vi "HFRR ADV v020 new software.vi"() -> ()   [LabVIEW 2025] (continued)
    n1953 = case shown="False" w2045 {
      frame False {
      }
      frame True {
      }
    }
    n1954 = case shown="True" w2035 {
      frame False {
        n1955 = property on="Password 2" class="Str"("Visible"=FALSE) -> ()  [unwired: 2 in, 2 out]
        n1956 = local write "Password 2"("" ("Password")) -> ()
      }
      frame True {
        n1957 = property on="Password 2" class="Str"("Visible"=TRUE) -> ()  [unwired: 2 in, 2 out]
        n1958 = Equal?(x="Password 2", y="HFRR1234") -> (x = y?=w2167:bool)
        n1959 = case shown="True" w2167 {
          tunnel: "Password 2" -> [w2170 _]
          frame False {
            n1960 = String Length(string=w2170) -> (length=w2171:i32)
            n1961 = Greater Than 0?(x=w2171) -> (x > 0?=w2169:bool)
            n1962 = case shown="False" w2169 {
              frame False {
                n1963 = property on="Password 2" class="Str"("Caption.Text"="Password (Advance Setting)") -> ()  [unwired: 2 in, 2 out]
              }
              frame True {
                n1964 = property on="Password 2" class="Str"("Caption.Text"="Incorrect Password!") -> ()  [unwired: 2 in, 2 out]
              }
            }
          }
          frame True {
            n1965 = local write "EDIT 2"(FALSE ("EDIT 2")) -> ()
            n1966 = local write "Password 2"("" ("Password")) -> ()
            n1967 = local write "Main Tab"(T2."Advance" ("Main Tab")) -> ()
            n1968 = local write "Main Dashboard Buttons"(T1."Advance" ("Main Dashboard Buttons")) -> ()
          }
        }
      }
    }
    n1969 = case shown="True" "Prog Uno" {
      frame False {
      }
      frame True {
        n1970 = stacked-sequence {
          frame #0 {
            n1971 = Delete(path (use dialog)=path "C:/LAB-IQ-NXT/UNOCOMPILE.bat" ("working directory")) -> ()  [unwired: 4 in, 3 out]
          }
          frame #1 {
            n1972 = local read "Com Port 1"() -> (w2632:refnum<visa-resource-name>)
            n1973 = Concatenate Strings("cmd.exe /c \"mode " ("command line"), w2632, ":1200,n,8,1\"\n" ("command line")) -> (w2637:string)
            n1974 = Concatenate Strings(w2637, "CD\\\nCD WinDucom\navrdude -C avrdude.conf -v -patmega328p -carduino -P" ("command line"), w2632, " -b115200 -D -Uflash:w:UNO_V20.hex:i\n" ("command line"), "\r") -> (w2639:string)
            "STR" <- w2639
            n1975 = call <vilib>:"Write Characters To File.vi"("append to file? (new file:F)"=FALSE, "character string"=w2639, "file path (dialog if empty)"=path "C:/LAB-IQ/UNOCOMPILE.bat" ("working directory")) -> ()  [unwired: 2 in, 1 out]
          }
          frame #2 {
            n1976 = disable-structure shown="Disabled" {
              frame Disabled {
                w2643 = "cmd.exe  /c \"C:\\LAB-IQ-NXT\\UNOCOMPILE.bat\"" ("string")
                n1977 = local write "Prog Uno"(FALSE ("run minimized? (F)")) -> ()
                n1978 = call <vilib>:"System Exec.vi"("expected output size  (4096)"=u32 65535, "run minimized? (F)"=FALSE, "wait until completion? (T)"=TRUE ("run minimized? (F)"), "working directory"=path "C:/LAB-IQ-NXT", "standard input"=w2643, "command line"=w2643) -> ("error out"=w2642:errorcluster, "standard output"=→"String 42":string)  [unwired: 2 in, 2 out]
                "error out 3" <- w2642
                n1979 = flat-sequence {
                  tunnel: w2642 -> [_]
                  frame #0 {
                  }
                }
              }
              frame Enabled {
              }
            }
          }
        }
      }
    }
    n1980 = case shown="\"ISO 12156\"" "TEST STANDARD" {
      tunnel: [2.0 ("Set Temp") 0.0 ("Set Temp") 2.0 ("Set Temp") 0.0 ("Set Temp")] -> w2036
      frame "ASTM D6079", Default {
        w2589 = 50.0 ("Hz")
        w2590 = 53.0 ("Set Rh")
        w2592 = 1.0 ("Set Strk")
        w2591 = 60.0 ("Set Temp")
        # "astm hide"
        n1981 = local write "NORMAL LOAD"(200.0 ("NORMAL LOAD")) -> ()
        n1982 = local write "Set Strk"(w2592) -> ()
        n1983 = local write "Set Hz"(w2589) -> ()
        n1984 = local write "Set Temp"(w2591) -> ()
        n1985 = local write "Set Rh"(w2590) -> ()
        n1986 = local write "test time"(75.0 ("test time")) -> ()
        n1987 = local write "Set Stroke:"(w2592) -> ()
        n1988 = local write "Set Humidity:"(w2590) -> ()
        n1989 = local write "Set Frequency:"(w2589) -> ()
        n1990 = local write "Set Temperature:"(w2591) -> ()
        "Test Standard" <- "ASTM D6079" ("Test Standard 2")
      }
      frame "ISO 12156" {
        n1991 = local write "Set Strk"(1.0 ("Set Strk")) -> ()
        n1992 = local write "NORMAL LOAD"(200.0 ("NORMAL LOAD")) -> ()
        n1993 = local write "Set Temp"(60.0 ("Set Temp")) -> ()
        n1994 = local write "test time"(75.0 ("test time")) -> ()
        n1995 = local write "Set Hz"(50.0 ("Hz")) -> ()
        n1996 = local write "Set Rh"(53.0 ("Set Rh")) -> ()
      }
      frame "CEC F-096-A-06" {
        n1997 = local write "Set Strk"(1.0 ("Set Strk")) -> ()
        n1998 = local write "NORMAL LOAD"(200.0 ("NORMAL LOAD")) -> ()
        n1999 = local write "Set Temp"(60.0 ("Set Temp")) -> ()
        n2000 = local write "test time"(75.0 ("test time")) -> ()
        n2001 = local write "Set Hz"(50.0 ("Hz")) -> ()
        n2002 = local write "Set Rh"(53.0 ("Set Rh")) -> ()
      }
      frame "Custom" {
      }
    }
    n2003 = case shown="True" "Prog Due" {
      frame False {
      }
      frame True {
        n2004 = stacked-sequence {
          frame #0 {
            n2005 = Delete(path (use dialog)=path "C:/LAB-IQ/DUECOMPILE.bat" ("working directory")) -> ()  [unwired: 4 in, 3 out]
          }
          frame #1 {
            n2006 = disable-structure shown="Disabled" {
              frame Disabled {
                n2007 = local read "visa due"() -> (w2614:string)
                n2008 = Concatenate Strings("cmd.exe /c \"mode " ("command line"), w2614, ":1200,n,8,1\"\n" ("command line")) -> (w2619:string)
                n2009 = Concatenate Strings(w2619, "CD\\\nCD WinDucom\nTIMEOUT 1\n bossac.exe -i -d --port=" ("command line"), w2614, " -U false -e -w -v -b DUE.bin -R\n" ("command line"), "\r") -> (w2621:string)
                "concatenated string 2" <- w2621
                n2010 = call <vilib>:"Write Characters To File.vi"("append to file? (new file:F)"=FALSE, "character string"=w2621, "file path (dialog if empty)"=path "C:/LAB-IQ-NXT/DUECOMPILE.bat" ("working directory")) -> ()  [unwired: 2 in, 1 out]
              }
              frame Enabled {
              }
            }
          }
          frame #2 {
            # "C:\\LAB-IQ-NXT\\DUECOMPILE.bat"
            n2011 = disable-structure shown="Disabled" {
              frame Disabled {
                w2626 = "cmd.exe  /c \"C:\\LAB-IQ-NXT\\DUECOMPILE.bat\"" ("string")
                n2012 = call <vilib>:"System Exec.vi"("expected output size  (4096)"=u32 65535, "run minimized? (F)"=FALSE, "wait until completion? (T)"=TRUE ("run minimized? (F)"), "working directory"=path "C:/LAB-IQ-NXT", "standard input"=w2626, "command line"=w2626) -> ("error out"=w2625:errorcluster, "standard output"=→"String 44":string)  [unwired: 2 in, 2 out]
                "error out 4" <- w2625
                n2013 = flat-sequence {
                  tunnel: w2625 -> [_]
                  frame #0 {
                  }
                }
              }
              frame Enabled {
              }
            }
            n2014 = local write "Prog Due"(FALSE ("Prog Due")) -> ()
          }
        }
      }
    }
    n2015 = Or(x=w2033, y=w2031) -> (x .or. y?=w2032:bool)
    n2016 = case shown="\"About\"" w2030 {
      tunnel: [T27."Acquire" ("Main Tab") T27."Compare Files" ("Main Tab") T27."About" ("Main Tab")] -> w2043
      frame "Acquire", Default {
      }
      frame "Compare Files" {
      }
      frame "About" {
      }
    }
    n2017 = Or(x=w2037, y="OPEN") -> (x .or. y?=w2038:bool)
    n2018 = case shown="True" w2038 {
      tunnel: w2037 -> [_ w2178]
      frame False {
      }
      frame True {
        n2019 = stacked-sequence {
          tunnel: w2178 -> [_ w2245 _ _]
          frame #0 {
            w2194 = "  " ("String 6")
            n2020 = local write "OPEN"(FALSE ("open")) -> ()
            n2021 = local read "string1 2"() -> (w2182:string)
            n2022 = local read "string1 3"() -> (w2181:string)
            n2023 = local read "string1 4"() -> (w2180:string)
            n2024 = property on="OPEN" class="Bool (strict)"("Visible"=FALSE) -> ()  [unwired: 2 in, 2 out]
            n2025 = local write "String 6"(w2194) -> ()
            n2026 = local write "String 7"(w2194) -> ()
            n2027 = local write "String 8"(w2194) -> ()
            n2028 = local write "String 12"(w2194) -> ()
            n2029 = local read "OK Button 16"() -> (w2179:bool)
            n2030 = String To Path(string=w2182) -> (path=w2190:path)
            n2031 = String To Path(string=w2181) -> (path=w2189:path)
            n2032 = String To Path(string=w2180) -> (path=w2188:path)
            n2033 = case shown="True" w2179 {
              tunnel: [w2195 w2196] -> w2183
              frame False {
                n2034 = local read "string1"() -> (w2195:string)
              }
              frame True {
                n2035 = local read "String Indicator 4"() -> (w2196:string)
              }
            }
            n2036 = Open/Create/Replace File "Open File"(file path (use dialog)=w2190) -> (refnum out=w2186:refnum<file>)  [unwired: 5 in, 2 out]
            n2037 = Open/Create/Replace File "Open File"(file path (use dialog)=w2189) -> (refnum out=w2185:refnum<file>)  [unwired: 5 in, 2 out]
            n2038 = Open/Create/Replace File "Open File"(file path (use dialog)=w2188) -> (refnum out=w2184:refnum<file>)  [unwired: 5 in, 2 out]
            n2039 = while {
              tunnel: w2186 -> [w2208]
              i -> [w2204]
              stop <- w2203 continue-if-true
              (unwired) TRUE ("line mode (F)")
              n2040 = Read from Text File "Read File"(file (use dialog)=w2208) -> (text=w2205:string)  [unwired: 3 in, 3 out]
              n2041 = local write "Numeric 11"(w2204) -> ()
              n2042 = String Length(string=w2205) -> (length=w2207:i32)
              n2043 = Greater?(x=w2207, y=1) -> (0:w2203:bool)
            }
            n2044 = while {
              tunnel: w2185 -> [w2214]
              i -> [w2210]
              stop <- w2209 continue-if-true
              (unwired) TRUE ("line mode (F)")
              n2045 = Read from Text File "Read File"(file (use dialog)=w2214) -> (text=w2211:string)  [unwired: 3 in, 3 out]
              n2046 = local write "Numeric 12"(w2210) -> ()
              n2047 = String Length(string=w2211) -> (length=w2213:i32)
              n2048 = Greater?(x=w2213, y=1) -> (0:w2209:bool)
            }
            n2049 = while {
              tunnel: w2184 -> [w2220]
              i -> [w2216]
              stop <- w2215 continue-if-true
              (unwired) TRUE ("line mode (F)")
              n2050 = Read from Text File "Read File"(file (use dialog)=w2220) -> (text=w2217:string)  [unwired: 3 in, 3 out]
              n2051 = local write "Numeric 13"(w2216) -> ()
              n2052 = String Length(string=w2217) -> (length=w2219:i32)
              n2053 = Greater?(x=w2219, y=1) -> (0:w2215:bool)
            }
            n2054 = String To Path(string=w2183) -> (path=w2191:path)
            n2055 = Open/Create/Replace File "Open File"(file path (use dialog)=w2191) -> (refnum out=w2187:refnum<file>)  [unwired: 5 in, 2 out]
            n2056 = while {
              tunnel: w2187 -> [w2202]
              i -> [w2198]
              stop <- w2197 continue-if-true
              (unwired) TRUE ("line mode (F)")
              n2057 = Read from Text File "Read File"(file (use dialog)=w2202) -> (text=w2199:string)  [unwired: 3 in, 3 out]
              n2058 = local write "Numeric 8"(w2198) -> ()
              n2059 = String Length(string=w2199) -> (length=w2201:i32)
              n2060 = Greater?(x=w2201, y=1) -> (0:w2197:bool)
            }
          }
          frame #1 {
            w2372 = FALSE ("ACTUAL   MERGE")
            # "Sample Temp"
            # "ECR"
            # "COF"
            # "Time\nCOF\nFF\nTemp"
            n2061 = case shown="True" w2245 {
              tunnel: [w2392 w2393] -> w2246
              frame False {
                n2062 = local read "string1"() -> (w2392:string)
              }
              frame True {
                n2063 = local read "String Indicator 4"() -> (w2393:string)
              }
            }
            n2064 = local read "string1 3"() -> (w2290:string)
            n2065 = String To Path(string=w2246) -> (path=w2377:path)
            n2066 = String To Path(string=w2290) -> (path=w2388:path)
            n2067 = local read "Numeric 12"() -> (w2374:i32)
            n2068 = local read "Numeric 8"() -> (w2376:i32)
            n2069 = local read "string1 2"() -> (w2291:string)
            n2070 = local read "string1 4"() -> (w2289:string)
            n2071 = Open/Create/Replace File "Open File"(file path (use dialog)=w2377) -> (refnum out=w2391:refnum<file>, error out=w2390:errorcluster)  [unwired: 5 in, 1 out]
            n2072 = Open/Create/Replace File "Open File"(file path (use dialog)=w2388) -> (refnum out=w2384:refnum<file>, error out=w2385:errorcluster)  [unwired: 5 in, 1 out]
            n2073 = for {
              N: w2376 -> [_]
              tunnel: w2391 -> [w2539]
              tunnel: w2390 -> [w2538]
              tunnel: [w2528] -> w2303 mode=indexing
              tunnel: [w2526] -> w2360 mode=indexing
              tunnel: [w2527] -> w2355 mode=indexing
              tunnel: w2372 -> [_]
              tunnel: [w2520] -> w2357 mode=indexing
              tunnel: [w2516] -> w2326 mode=indexing
              tunnel: [w2512] -> w2301 mode=indexing
              tunnel: [w2508] -> w2282 mode=indexing
              tunnel: [w2503] -> w2242 mode=indexing
              (unwired) TRUE ("line mode (F)")
              # "freq"
              # "Stroke"
              # "Time"
              # "CoF"
              # "Humidity"
              # "Temp"
              # "Air Temp"
              # "ECR"
              n2074 = Read from Text File "Read File"(file (use dialog)=w2539, error in=w2538) -> (text=w2504:string)  [unwired: 2 in, 3 out]
              n2075 = local write "String 6"(w2504) -> ()
              n2076 = String Subset(string=w2504, offset (0)=0, length (rest)=14 ("length (rest)")) -> (substring=w2532:string)
              n2077 = String Subset(string=w2504, offset (0)=35, length (rest)=9 ("length (rest)")) -> (substring=w2529:string)
              n2078 = String Subset(string=w2504, offset (0)=15, length (rest)=9 ("length (rest)")) -> (substring=w2535:string)
              n2079 = Fract/Exp String To Number(string=w2532) -> (number=w2528:dbl)  [unwired: 3 in, 1 out]
              n2080 = Fract/Exp String To Number(string=w2529) -> (number=w2527:dbl)  [unwired: 3 in, 1 out]
              n2081 = Fract/Exp String To Number(string=w2535) -> (number=w2526:dbl)  [unwired: 3 in, 1 out]
              n2082 = String Subset(string=w2504, offset (0)=85, length (rest)=9 ("length (rest)")) -> (substring=w2505:string)
              n2083 = String Subset(string=w2504, offset (0)=25, length (rest)=9 ("length (rest)")) -> (substring=w2511:string)
              n2084 = String Subset(string=w2504, offset (0)=55, length (rest)=9 ("length (rest)")) -> (substring=w2513:string)
              n2085 = String Subset(string=w2504, offset (0)=45, length (rest)=9 ("length (rest)")) -> (substring=w2519:string)
              n2086 = String Subset(string=w2504, offset (0)=65, length (rest)=9 ("length (rest)")) -> (substring=w2525:string)
              n2087 = Fract/Exp String To Number(string=w2511) -> (number=w2508:dbl)  [unwired: 3 in, 1 out]
              n2088 = Fract/Exp String To Number(string=w2505) -> (number=w2503:dbl)  [unwired: 3 in, 1 out]
              n2089 = Fract/Exp String To Number(string=w2513) -> (number=w2512:dbl)  [unwired: 3 in, 1 out]
              n2090 = Fract/Exp String To Number(string=w2519) -> (number=w2516:dbl)  [unwired: 3 in, 1 out]
              n2091 = Fract/Exp String To Number(string=w2525) -> (number=w2522:dbl)  [unwired: 3 in, 1 out]
              n2092 = Add(x=w2522, y=0.0) -> (x+y=w2520:dbl)
            }
            n2093 = for {
              N: w2374 -> [_]
              tunnel: w2385 -> [w2465]
              tunnel: w2384 -> [w2464]
              tunnel: [w2454] -> w2343 mode=indexing
              tunnel: [w2452] -> w2341 mode=indexing
              tunnel: [w2453] -> w2337 mode=indexing
              tunnel: w2372 -> [_]
              tunnel: [w2446] -> w2339 mode=indexing
              tunnel: [w2442] -> w2321 mode=indexing
              tunnel: [w2438] -> w2297 mode=indexing
              tunnel: [w2435] -> w2278 mode=indexing
              tunnel: [w2431] -> w2237 mode=indexing
              (unwired) 9 ("length (rest)")
              (unwired) 9 ("length (rest)")
              (unwired) TRUE ("line mode (F)")
              n2094 = Read from Text File "Read File"(file (use dialog)=w2464, error in=w2465) -> (text=w2432:string)  [unwired: 2 in, 3 out]
              n2095 = local write "String 8"(w2432) -> ()
              n2096 = String Subset(string=w2432, offset (0)=85) -> (substring=w2434:string)  [unwired: 1 in]
              n2097 = String Subset(string=w2432, offset (0)=35, length (rest)=9 ("length (rest)")) -> (substring=w2455:string)
              n2098 = String Subset(string=w2432, offset (0)=55, length (rest)=9 ("length (rest)")) -> (substring=w2440:string)
              n2099 = String Subset(string=w2432, offset (0)=25) -> (substring=w2436:string)  [unwired: 1 in]
              n2100 = String Subset(string=w2432, offset (0)=15, length (rest)=9 ("length (rest)")) -> (substring=w2461:string)
              n2101 = String Subset(string=w2432, offset (0)=0, length (rest)=14 ("length (rest)")) -> (substring=w2458:string)
              n2102 = String Subset(string=w2432, offset (0)=45, length (rest)=9 ("length (rest)")) -> (substring=w2445:string)
              n2103 = String Subset(string=w2432, offset (0)=65, length (rest)=9 ("length (rest)")) -> (substring=w2451:string)
              n2104 = Fract/Exp String To Number(string=w2434) -> (number=w2431:dbl)  [unwired: 3 in, 1 out]
              n2105 = Fract/Exp String To Number(string=w2455) -> (number=w2453:dbl)  [unwired: 3 in, 1 out]
              n2106 = Fract/Exp String To Number(string=w2440) -> (number=w2438:dbl)  [unwired: 3 in, 1 out]
              n2107 = Fract/Exp String To Number(string=w2436) -> (number=w2435:dbl)  [unwired: 3 in, 1 out]
              n2108 = Fract/Exp String To Number(string=w2461) -> (number=w2452:dbl)  [unwired: 3 in, 1 out]
              n2109 = Fract/Exp String To Number(string=w2458) -> (number=w2454:dbl)  [unwired: 3 in, 1 out]
              n2110 = Fract/Exp String To Number(string=w2445) -> (number=w2442:dbl)  [unwired: 3 in, 1 out]
              n2111 = Fract/Exp String To Number(string=w2451) -> (number=w2448:dbl)  [unwired: 3 in, 1 out]
              n2112 = Add(x=w2448, y=0.0) -> (x+y=w2446:dbl)
            }
            n2113 = String To Path(string=w2291) -> (path=w2389:path)
            n2114 = String To Path(string=w2289) -> (path=w2383:path)
            n2115 = local read "Numeric 11"() -> (w2373:i32)
            n2116 = local read "Numeric 13"() -> (w2375:i32)
            n2117 = Open/Create/Replace File "Open File"(file path (use dialog)=w2389) -> (refnum out=w2387:refnum<file>, error out=w2386:errorcluster)  [unwired: 5 in, 1 out]
            n2118 = Open/Create/Replace File "Open File"(file path (use dialog)=w2383) -> (refnum out=w2382:refnum<file>, error out=w2381:errorcluster)  [unwired: 5 in, 1 out]
            n2119 = for {
              N: w2373 -> [_]
              tunnel: w2387 -> [w2502]
              tunnel: w2386 -> [w2501]
              tunnel: [w2491] -> w2353 mode=indexing
              tunnel: [w2489] -> w2351 mode=indexing
              tunnel: [w2490] -> w2346 mode=indexing
              tunnel: w2372 -> [_]
              tunnel: [w2483] -> w2348 mode=indexing
              tunnel: [w2479] -> w2324 mode=indexing
              tunnel: [w2475] -> w2299 mode=indexing
              tunnel: [w2471] -> w2280 mode=indexing
              tunnel: [w2466] -> w2238 mode=indexing
              (unwired) TRUE ("line mode (F)")
              n2120 = Read from Text File "Read File"(file (use dialog)=w2502, error in=w2501) -> (text=w2467:string)  [unwired: 2 in, 3 out]
              n2121 = local write "String 7"(w2467) -> ()
              n2122 = String Subset(string=w2467, offset (0)=85, length (rest)=9 ("length (rest)")) -> (substring=w2470:string)
              n2123 = String Subset(string=w2467, offset (0)=35, length (rest)=9 ("length (rest)")) -> (substring=w2492:string)
              n2124 = String Subset(string=w2467, offset (0)=55, length (rest)=9 ("length (rest)")) -> (substring=w2478:string)
              n2125 = String Subset(string=w2467, offset (0)=25, length (rest)=9 ("length (rest)")) -> (substring=w2472:string)
              n2126 = String Subset(string=w2467, offset (0)=45, length (rest)=9 ("length (rest)")) -> (substring=w2480:string)
              n2127 = String Subset(string=w2467, offset (0)=0, length (rest)=14 ("length (rest)")) -> (substring=w2495:string)
              n2128 = String Subset(string=w2467, offset (0)=15, length (rest)=9 ("length (rest)")) -> (substring=w2498:string)
              n2129 = String Subset(string=w2467, offset (0)=65, length (rest)=9 ("length (rest)")) -> (substring=w2484:string)
              n2130 = Fract/Exp String To Number(string=w2470) -> (number=w2466:dbl)  [unwired: 3 in, 1 out]
              n2131 = Fract/Exp String To Number(string=w2492) -> (number=w2490:dbl)  [unwired: 3 in, 1 out]
              n2132 = Fract/Exp String To Number(string=w2478) -> (number=w2475:dbl)  [unwired: 3 in, 1 out]
              n2133 = Fract/Exp String To Number(string=w2472) -> (number=w2471:dbl)  [unwired: 3 in, 1 out]
              n2134 = Fract/Exp String To Number(string=w2480) -> (number=w2479:dbl)  [unwired: 3 in, 1 out]
              n2135 = Fract/Exp String To Number(string=w2495) -> (number=w2491:dbl)  [unwired: 3 in, 1 out]
              n2136 = Fract/Exp String To Number(string=w2498) -> (number=w2489:dbl)  [unwired: 3 in, 1 out]
              n2137 = Fract/Exp String To Number(string=w2484) -> (number=w2487:dbl)  [unwired: 3 in, 1 out]
              n2138 = Add(x=w2487, y=0.0) -> (x+y=w2483:dbl)
            }
            n2139 = for {
              N: w2375 -> [_]
              tunnel: w2382 -> [w2430]
              tunnel: w2381 -> [w2429]
              tunnel: [w2419] -> w2335 mode=indexing
              tunnel: [w2418] -> w2328 mode=indexing
              tunnel: w2372 -> [_]
              tunnel: [w2407] -> w2333 mode=indexing
              tunnel: [w2412] -> w2330 mode=indexing
              tunnel: [w2408] -> w2320 mode=indexing
              tunnel: [w2403] -> w2295 mode=indexing
              tunnel: [w2399] -> w2276 mode=indexing
              tunnel: [w2394] -> w2236 mode=indexing
              (unwired) 1.0 ("x")
              (unwired) TRUE ("line mode (F)")
              n2140 = Read from Text File "Read File"(file (use dialog)=w2430, error in=w2429) -> (text=w2395:string)  [unwired: 2 in, 3 out]
              n2141 = local write "String 12"(w2395) -> ()
              n2142 = String Subset(string=w2395, offset (0)=85, length (rest)=9 ("length (rest)")) -> (substring=w2397:string)
              n2143 = String Subset(string=w2395, offset (0)=35, length (rest)=9 ("length (rest)")) -> (substring=w2420:string)
              n2144 = String Subset(string=w2395, offset (0)=55, length (rest)=9 ("length (rest)")) -> (substring=w2405:string)
              n2145 = String Subset(string=w2395, offset (0)=25, length (rest)=9 ("length (rest)")) -> (substring=w2401:string)
              n2146 = String Subset(string=w2395, offset (0)=45, length (rest)=9 ("length (rest)")) -> (substring=w2410:string)
              n2147 = String Subset(string=w2395, offset (0)=15, length (rest)=9 ("length (rest)")) -> (substring=w2426:string)
              n2148 = String Subset(string=w2395, offset (0)=0, length (rest)=14 ("length (rest)")) -> (substring=w2423:string)
              n2149 = String Subset(string=w2395, offset (0)=65, length (rest)=9 ("length (rest)")) -> (substring=w2413:string)
              n2150 = Fract/Exp String To Number(string=w2397) -> (number=w2394:dbl)  [unwired: 3 in, 1 out]
              n2151 = Fract/Exp String To Number(string=w2420) -> (number=w2418:dbl)  [unwired: 3 in, 1 out]
              n2152 = Fract/Exp String To Number(string=w2405) -> (number=w2403:dbl)  [unwired: 3 in, 1 out]
              n2153 = Fract/Exp String To Number(string=w2401) -> (number=w2399:dbl)  [unwired: 3 in, 1 out]
              n2154 = Fract/Exp String To Number(string=w2410) -> (number=w2408:dbl)  [unwired: 3 in, 1 out]
              n2155 = Fract/Exp String To Number(string=w2426) -> (number=w2407:dbl)  [unwired: 3 in, 1 out]
              n2156 = Fract/Exp String To Number(string=w2423) -> (number=w2419:dbl)  [unwired: 3 in, 1 out]
              n2157 = Fract/Exp String To Number(string=w2413) -> (number=w2416:dbl)  [unwired: 3 in, 1 out]
              n2158 = Add(x=w2416, y=0.0) -> (x+y=w2412:dbl)
            }
            n2159 = Delete From Array(array=w2278, index=0) -> (array with subset deleted=w2251:dbl[])  [unwired: 1 in, 1 out]
            n2160 = Delete From Array(array=w2341, index=0) -> (array with subset deleted=w2314:dbl[])  [unwired: 1 in, 1 out]
            n2161 = Delete From Array(array=w2321, index=0) -> (array with subset deleted=w2309:dbl[])  [unwired: 1 in, 1 out]
            n2162 = Delete From Array(array=w2339, index=0) -> (array with subset deleted=w2340:dbl[])  [unwired: 1 in, 1 out]
            n2163 = call-poly <vilib>:"Mean.vi"("X"=w2251) -> ("mean"=→"КОФ2 4":dbl)  [unwired: 1 out]
            n2164 = call-poly <vilib>:"Mean.vi"("X"=w2314) -> ("mean"=→"КОФ3":dbl)  [unwired: 1 out]
            n2165 = call-poly <vilib>:"Mean.vi"("X"=w2309) -> ("mean"=→"CP3":dbl)  [unwired: 1 out]
            n2166 = Delete From Array(array=w2303, index=0) -> (array with subset deleted=w2230:dbl[])  [unwired: 1 in, 1 out]
            n2167 = Delete From Array(array=w2242, index=0) -> (array with subset deleted=w2229:dbl[])  [unwired: 1 in, 1 out]
            n2168 = Delete From Array(array=w2282, index=0) -> (array with subset deleted=w2253:dbl[])  [unwired: 1 in, 1 out]
            n2169 = Delete From Array(array=w2360, index=0) -> (array with subset deleted=w2315:dbl[])  [unwired: 1 in, 1 out]
            n2170 = Delete From Array(array=w2326, index=0) -> (array with subset deleted=w2311:dbl[])  [unwired: 1 in, 1 out]
            "array w/ subset deleted" <- w2311
            n2171 = Delete From Array(array=w2357, index=0) -> (array with subset deleted=w2358:dbl[])  [unwired: 1 in, 1 out]
            n2172 = call-poly <vilib>:"Mean.vi"("X"=w2253) -> ("mean"=→"КОФ2 2":dbl)  [unwired: 1 out]
            n2173 = call-poly <vilib>:"Mean.vi"("X"=w2315) -> ("mean"=→"КОФ1":dbl)  [unwired: 1 out]
            n2174 = Bundle "Bundle"(w2230, w2229) -> (w2235:cluster{dbl[], dbl[]})  [unwired: 1 in]
            n2175 = Bundle "Bundle"(w2230, w2358) -> (w2222:cluster{dbl[], dbl[]})  [unwired: 1 in]
            n2176 = Delete From Array(array=w2237, index=0) -> (array with subset deleted=w2225:dbl[])  [unwired: 1 in, 1 out]
            n2177 = Delete From Array(array=w2238, index=0) -> (array with subset deleted=w2227:dbl[])  [unwired: 1 in, 1 out]
            n2178 = Delete From Array(array=w2348, index=0) -> (array with subset deleted=w2349:dbl[])  [unwired: 1 in, 1 out]
            n2179 = Delete From Array(array=w2236, index=0) -> (array with subset deleted=w2223:dbl[])  [unwired: 1 in, 1 out]
            n2180 = Delete From Array(array=w2330, index=0) -> (array with subset deleted=w2331:dbl[])  [unwired: 1 in, 1 out]
            n2181 = Delete From Array(array=w2355, index=0) -> (array with subset deleted=w2261:dbl[])  [unwired: 1 in, 1 out]
            n2182 = Delete From Array(array=w2301, index=0) -> (array with subset deleted=w2257:dbl[])  [unwired: 1 in, 1 out]
            n2183 = Delete From Array(array=w2337, index=0) -> (array with subset deleted=w2259:dbl[])  [unwired: 1 in, 1 out]
            n2184 = Delete From Array(array=w2297, index=0) -> (array with subset deleted=w2255:dbl[])  [unwired: 1 in, 1 out]
            n2185 = Delete From Array(array=w2346, index=0) -> (array with subset deleted=w2260:dbl[])  [unwired: 1 in, 1 out]
            n2186 = Delete From Array(array=w2299, index=0) -> (array with subset deleted=w2256:dbl[])  [unwired: 1 in, 1 out]
            n2187 = Delete From Array(array=w2280, index=0) -> (array with subset deleted=w2252:dbl[])  [unwired: 1 in, 1 out]
            n2188 = Delete From Array(array=w2324, index=0) -> (array with subset deleted=w2310:dbl[])  [unwired: 1 in, 1 out]
            n2189 = Delete From Array(array=w2351, index=0) -> (array with subset deleted=w2312:dbl[])  [unwired: 1 in, 1 out]
            n2190 = Delete From Array(array=w2328, index=0) -> (array with subset deleted=w2258:dbl[])  [unwired: 1 in, 1 out]
            n2191 = Delete From Array(array=w2295, index=0) -> (array with subset deleted=w2254:dbl[])  [unwired: 1 in, 1 out]
            n2192 = Delete From Array(array=w2276, index=0) -> (array with subset deleted=w2250:dbl[])  [unwired: 1 in, 1 out]
            n2193 = Delete From Array(array=w2320, index=0) -> (array with subset deleted=w2308:dbl[])  [unwired: 1 in, 1 out]
            n2194 = Delete From Array(array=w2333, index=0) -> (array with subset deleted=w2313:dbl[])  [unwired: 1 in, 1 out]
            n2195 = Delete From Array(array=w2343, index=0) -> (array with subset deleted=w2226:dbl[])  [unwired: 1 in, 1 out]
            n2196 = Delete From Array(array=w2353, index=0) -> (array with subset deleted=w2228:dbl[])  [unwired: 1 in, 1 out]
            n2197 = Delete From Array(array=w2335, index=0) -> (array with subset deleted=w2224:dbl[])  [unwired: 1 in, 1 out]
            n2198 = Bundle "Bundle"(w2230, w2261) -> (w2248:cluster{dbl[], dbl[]})  [unwired: 1 in]
            n2199 = Bundle "Bundle"(w2230, w2315) -> (w2249:cluster{dbl[], dbl[]})  [unwired: 1 in]
            n2200 = Bundle "Bundle"(w2261, w2257) -> (w2263:cluster{dbl[], dbl[]})  [unwired: 1 in]
            n2201 = Bundle "Bundle"(w2226, w2225) -> (w2233:cluster{dbl[], dbl[]})  [unwired: 1 in]
            n2202 = Bundle "Bundle"(w2259, w2255) -> (w2265:cluster{dbl[], dbl[]})  [unwired: 1 in]
            n2203 = Bundle "Bundle"(w2226, w2259) -> (w2369:cluster{dbl[], dbl[]})  [unwired: 1 in]
            n2204 = Bundle "Bundle"(w2226, w2255) -> (w2293:cluster{dbl[], dbl[]})  [unwired: 1 in]
            n2205 = Bundle "Bundle"(w2226, w2314) -> (w2379:cluster{dbl[], dbl[]})  [unwired: 1 in]
            n2206 = Bundle "Bundle"(w2226, w2309) -> (w2317:cluster{dbl[], dbl[]})  [unwired: 1 in]
            n2207 = Bundle "Bundle"(w2226, w2340) -> (w2364:cluster{dbl[], dbl[]})  [unwired: 1 in]
            n2208 = Bundle "Bundle"(w2260, w2256) -> (w2264:cluster{dbl[], dbl[]})  [unwired: 1 in]
            n2209 = Bundle "Bundle"(w2228, w2227) -> (w2234:cluster{dbl[], dbl[]})  [unwired: 1 in]
            n2210 = Bundle "Bundle"(w2228, w2260) -> (w2371:cluster{dbl[], dbl[]})  [unwired: 1 in]
            n2211 = Bundle "Bundle"(w2228, w2256) -> (w2294:cluster{dbl[], dbl[]})  [unwired: 1 in]
            n2212 = Bundle "Bundle"(w2228, w2310) -> (w2318:cluster{dbl[], dbl[]})  [unwired: 1 in]
            n2213 = Bundle "Bundle"(w2228, w2312) -> (w2380:cluster{dbl[], dbl[]})  [unwired: 1 in]
            n2214 = Bundle "Bundle"(w2228, w2349) -> (w2362:cluster{dbl[], dbl[]})  [unwired: 1 in]
            n2215 = Bundle "Bundle"(w2258, w2254) -> (w2266:cluster{dbl[], dbl[]})  [unwired: 1 in]
            n2216 = Bundle "Bundle"(w2224, w2223) -> (w2232:cluster{dbl[], dbl[]})  [unwired: 1 in]
            n2217 = Bundle "Bundle"(w2224, w2258) -> (w2370:cluster{dbl[], dbl[]})  [unwired: 1 in]
            n2218 = Bundle "Bundle"(w2224, w2254) -> (w2292:cluster{dbl[], dbl[]})  [unwired: 1 in]
            n2219 = Bundle "Bundle"(w2224, w2308) -> (w2316:cluster{dbl[], dbl[]})  [unwired: 1 in]
            n2220 = Bundle "Bundle"(w2224, w2313) -> (w2378:cluster{dbl[], dbl[]})  [unwired: 1 in]
            n2221 = Bundle "Bundle"(w2224, w2331) -> (w2363:cluster{dbl[], dbl[]})  [unwired: 1 in]
            n2222 = call-poly <vilib>:"Mean.vi"("X"=w2311) -> ("mean"=→"CP1":dbl)  [unwired: 1 out]
            n2223 = call-poly <vilib>:"Mean.vi"("X"=w2252) -> ("mean"=→"КОФ2 3":dbl)  [unwired: 1 out]
            n2224 = call-poly <vilib>:"Mean.vi"("X"=w2310) -> ("mean"=→"CP2":dbl)  [unwired: 1 out]
            n2225 = call-poly <vilib>:"Mean.vi"("X"=w2312) -> ("mean"=→"КОФ2":dbl)  [unwired: 1 out]
            n2226 = call-poly <vilib>:"Mean.vi"("X"=w2250) -> ("mean"=→"КОФ2 5":dbl)  [unwired: 1 out]
            n2227 = call-poly <vilib>:"Mean.vi"("X"=w2308) -> ("mean"=→"CP4":dbl)  [unwired: 1 out]
            n2228 = call-poly <vilib>:"Mean.vi"("X"=w2313) -> ("mean"=→"КОФ4":dbl)  [unwired: 1 out]
            n2229 = Bundle "Bundle"(w2230, w2257) -> (w2221:cluster{dbl[], dbl[]})  [unwired: 1 in]
            n2230 = Bundle "Bundle"(w2230, w2311) -> (w2244:cluster{dbl[], dbl[]})  [unwired: 1 in]
            n2231 = Build Array "Build Array"(w2221, w2244) -> (w2247:cluster{dbl[], dbl[]}[])
            "XY Graph 17" <- w2247
            n2232 = Build Array "Build Array"(w2235, w2234, w2233, w2232) -> (→"Frequency ( Hz )":cluster{dbl[], dbl[]}[])
            n2233 = Build Array "Build Array"(w2263, w2264, w2265, w2266) -> (→"Air Temp ( °C ) vs Humidity ( % RH )":cluster{dbl[], dbl[]}[])
            n2234 = Build Array "Build Array"(w2248, w2371, w2369, w2370) -> (→"Air Temperature  ( °C )":cluster{dbl[], dbl[]}[])
            n2235 = Build Array "Build Array"(w2221, w2294, w2293, w2292) -> (→"Humidity ( %RH )":cluster{dbl[], dbl[]}[])
            n2236 = Build Array "Build Array"(w2249, w2380, w2379, w2378) -> (→"Coefficient Of Friction":cluster{dbl[], dbl[]}[])
            n2237 = Build Array "Build Array"(w2244, w2318, w2317, w2316) -> (→"Sample Temperature ( °C )":cluster{dbl[], dbl[]}[])
            n2238 = Build Array "Build Array"(w2222, w2362, w2364, w2363) -> (→"XY Graph 13":cluster{dbl[], dbl[]}[])
            n2239 = Bundle "Bundle"(w2230, w2253) -> (w2275:cluster{dbl[], dbl[]})  [unwired: 1 in]
            n2240 = Bundle "Bundle"(w2226, w2251) -> (w2273:cluster{dbl[], dbl[]})  [unwired: 1 in]
            n2241 = Bundle "Bundle"(w2228, w2252) -> (w2274:cluster{dbl[], dbl[]})  [unwired: 1 in]
            n2242 = Bundle "Bundle"(w2224, w2250) -> (w2272:cluster{dbl[], dbl[]})  [unwired: 1 in]
            n2243 = Build Array "Build Array"(w2275, w2274, w2273, w2272) -> (→"Stroke ( mm )":cluster{dbl[], dbl[]}[])
            n2244 = local write "XY Graph 16"(w2247) -> ()
          }
          frame #2 {
          }
          frame #3 {
            n2245 = local write "Numeric 8"(0 ("Numeric 8")) -> ()
            n2246 = local write "Numeric 11"(0 ("Numeric 11")) -> ()
            n2247 = local write "Numeric 12"(0 ("Numeric 12")) -> ()
            n2248 = local write "Numeric 13"(0 ("Numeric 13")) -> ()
            n2249 = property on="OPEN" class="Bool (strict)"("Visible"=TRUE) -> ()  [unwired: 2 in, 2 out]
            n2250 = local read "String Control 2"() -> (w2547:string)
            n2251 = local read "String Control 4"() -> (w2546:string)
            n2252 = local read "String Control 6"() -> (w2545:string)
            n2253 = local read "String Control 8"() -> (w2544:string)
            n2254 = Match Pattern(string=w2547, regular expression="Samples / cycle :- ") -> (after substring=w2561:string)  [unwired: 1 in, 3 out]
            n2255 = Match Pattern(string=w2547, regular expression="Frequency :- ") -> (after substring=w2580:string)  [unwired: 1 in, 3 out]
            n2256 = Match Pattern(string=w2546, regular expression="Samples / cycle :- ") -> (after substring=w2557:string)  [unwired: 1 in, 3 out]
            n2257 = Match Pattern(string=w2546, regular expression="Frequency :- ") -> (after substring=w2575:string)  [unwired: 1 in, 3 out]
            n2258 = Match Pattern(string=w2545, regular expression="Samples / cycle :- ") -> (after substring=w2553:string)  [unwired: 1 in, 3 out]
            n2259 = Match Pattern(string=w2545, regular expression="Frequency :- ") -> (after substring=w2570:string)  [unwired: 1 in, 3 out]
            n2260 = Match Pattern(string=w2544, regular expression="Samples / cycle :- ") -> (after substring=w2549:string)  [unwired: 1 in, 3 out]
            n2261 = Match Pattern(string=w2544, regular expression="Frequency :- ") -> (after substring=w2565:string)  [unwired: 1 in, 3 out]
            n2262 = String Subset(string=w2561, length (rest)=6 ("length (rest)")) -> (substring=w2563:string)  [unwired: 1 in]
            n2263 = String Subset(string=w2580, length (rest)=9 ("length (rest)")) -> (substring=w2582:string)  [unwired: 1 in]
            n2264 = String Subset(string=w2557, length (rest)=6 ("length (rest)")) -> (substring=w2559:string)  [unwired: 1 in]
            n2265 = String Subset(string=w2575, length (rest)=9 ("length (rest)")) -> (substring=w2577:string)  [unwired: 1 in]
            n2266 = String Subset(string=w2553, length (rest)=6 ("length (rest)")) -> (substring=w2555:string)  [unwired: 1 in]
            n2267 = String Subset(string=w2570, length (rest)=9 ("length (rest)")) -> (substring=w2572:string)  [unwired: 1 in]
            n2268 = String Subset(string=w2549, length (rest)=6 ("length (rest)")) -> (substring=w2551:string)  [unwired: 1 in]
            n2269 = String Subset(string=w2565, length (rest)=9 ("length (rest)")) -> (substring=w2567:string)  [unwired: 1 in]
            n2270 = Fract/Exp String To Number(string=w2563) -> (number=w2543:dbl)  [unwired: 3 in, 1 out]
            n2271 = Fract/Exp String To Number(string=w2582) -> (number=w2583:dbl)  [unwired: 3 in, 1 out]
            n2272 = Fract/Exp String To Number(string=w2559) -> (number=w2542:dbl)  [unwired: 3 in, 1 out]
            n2273 = Fract/Exp String To Number(string=w2577) -> (number=w2578:dbl)  [unwired: 3 in, 1 out]
            n2274 = Fract/Exp String To Number(string=w2555) -> (number=w2541:dbl)  [unwired: 3 in, 1 out]
            n2275 = Fract/Exp String To Number(string=w2572) -> (number=w2573:dbl)  [unwired: 3 in, 1 out]
            n2276 = Fract/Exp String To Number(string=w2551) -> (number=w2540:dbl)  [unwired: 3 in, 1 out]
            n2277 = Fract/Exp String To Number(string=w2567) -> (number=w2568:dbl)  [unwired: 3 in, 1 out]
            n2278 = local write "sample1"(w2543) -> ()
            n2279 = local write "freq1"(w2583) -> ()
            n2280 = local write "sample2"(w2542) -> ()
            n2281 = local write "freq2"(w2578) -> ()
            n2282 = local write "sample3"(w2541) -> ()
            n2283 = local write "freq3"(w2573) -> ()
            n2284 = local write "sample4"(w2540) -> ()
            n2285 = local write "freq 4"(w2568) -> ()
          }
        }
      }
    }
    n2286 = case shown="True" w2032 {
      selector: w2032 -> [_ w2160]
      frame False {
      }
      frame True {
        n2287 = Not(x=w2160) -> (.not. x?=w2156:bool)
        n2288 = local write "service 3"(w2156) -> ()
        n2289 = local write "OPEN 6"(w2156) -> ()
        n2290 = call <vilib>:"System Exec.vi"("wait until completion? (T)"=TRUE, "command line"="C:\\LAB-IQ\\Scar View.exe") -> ("error out"=→"error out 5":errorcluster)  [unwired: 6 in, 3 out]
      }
    }
    n2291 = case shown="\"Acquire\", Default" w2043 {
      frame "Acquire", Default {
        w3056 = 0.2 ("y")
        w3061 = 1.0 ("y")
        w3062 = 0.8 ("y")
        # "Elapsed time\ncof\nstroke\nAir temp\nTemp\nHumidity"
        n2292 = disable-structure shown="Disabled" {
          frame Disabled {
            n2293 = local read "Flag"() -> (w3079:dbl)
            n2294 = local read "RUN"() -> (w3076:bool)
            n2295 = Not(x=w3076) -> (.not. x?=w3075:bool)
            n2296 = Equal?(x=w3079, y=10.0) -> (x = y?=w3077:bool)
            n2297 = And(x=w3077, y=w3075) -> (x .and. y?=w3074:bool)
            n2298 = case shown="True" w3074 {
              frame False {
              }
              frame True {
                w3080 = FALSE ("Heater Button")
                n2299 = local write "Humidity"(w3080) -> ()
                n2300 = local write "Heater Button"(w3080) -> ()
              }
            }
          }
          frame Enabled {
          }
        }
        n2301 = disable-structure shown="Disabled" {
          frame Disabled {
            n2302 = case shown="True" {
              selector: _ -> [_ _]
              frame False {
              }
              frame True {
                w3171 = TRUE ("Heater")
                n2303 = local write "Humidity"(w3171) -> ()
                n2304 = local write "Heater Button"(w3171) -> ()
                n2305 = local read "TEST STANDARD"() -> (w3174:T3)
                n2306 = local read "TEST STANDARD"() -> (w3169:T3)
                n2307 = Equal?(x=w3174, y=enum16{"ASTM D6079", "ISO 12156", "Custom"}."ISO 12156" ("Test Standard")) -> (x = y?=w3172:bool)
                n2308 = Equal?(x=w3169, y=enum16{"ASTM D6079", "ISO 12156", "Custom"}."ASTM D6079" ("Test Standard")) -> (x = y?=w3168:bool)
                n2309 = case shown="True" w3172 {
                  frame False {
                  }
                  frame True {
                    n2310 = local write "Heater"(TRUE ("Heater")) -> ()
                    n2311 = local write "airtempflg"(FALSE ("airtempflg")) -> ()
                  }
                }
                n2312 = case shown="True" w3168 {
                  frame False {
                  }
                  frame True {
                    n2313 = local write "Heater"(FALSE ("Heater")) -> ()
                    n2314 = local write "airtempflg"(TRUE ("airtempflg")) -> ()
                  }
                }
              }
            }
          }
          frame Enabled {
          }
        }
        n2315 = stacked-sequence {
          frame #0 {
            n2316 = case shown="True" "RST FF" {
              frame False {
              }
              frame True {
                w3237 = 0.0 ("X Scale.Range:Maximum")
                n2317 = property on="Frictional Force ( N )" class="WFChart (strict)"("XScale.Maximum"=600.0 ("X Scale.Range:Maximum"), "XScale.Minimum"=w3237, "YScale.Maximum"=10.0 ("Y Scale.Range:Maximum"), "YScale.Minimum"=w3237) -> ()  [unwired: 2 in, 2 out]
              }
            }
          }
          frame #1 {
            n2318 = case shown="True" "RST TEMP" {
              frame False {
              }
              frame True {
                n2319 = property on="Temperature ( Deg C )" class="WFChart (strict)"("XScale.Minimum"=0.0 ("X Scale.Range:Minimum"), "XScale.Maximum"=600.0 ("X Scale.Range:Maximum"), "YScale.Minimum"=0.0 ("Y Scale.Range:Minimum"), "YScale.Maximum"=100.0 ("Y Scale.Range:Maximum")) -> ()  [unwired: 2 in, 2 out]
              }
            }
          }
          frame #2 {
            n2320 = case shown="True" "RSTCOF" {
              frame False {
              }
              frame True {
                n2321 = property on="Coefficient of Friction" class="WFChart (strict)"("XScale.Minimum"=0.0 ("X Scale.Range:Minimum"), "XScale.Maximum"=600.0 ("X Scale.Range:Maximum"), "YScale.Maximum"=1.0 ("X Scale.Range:Minimum"), "YScale.Minimum"=0.0 ("X Scale.Range:Minimum")) -> ()  [unwired: 2 in, 2 out]
              }
            }
          }
          frame #3 {
            n2322 = case shown="True" "RSTCOF 2" {
              frame False {
              }
              frame True {
                (unwired) 100.0 ("Y Scale.Range:Maximum")
                (unwired) 0.0 ("Y Scale.Range:Minimum")
                (unwired) 600.0 ("X Scale.Range:Maximum")
                (unwired) 0.0 ("X Scale.Range:Minimum")
              }
            }
          }
          frame #4 {
            n2323 = case shown="True" "RSTCOF 3" {
              frame False {
              }
              frame True {
                n2324 = property on="Electrical Contact Resistance ( % )" class="WFChart (strict)"("XScale.Minimum"=0.0 ("X Scale.Range:Minimum"), "XScale.Maximum"=600.0 ("X Scale.Range:Maximum"), "YScale.Minimum"=0.0 ("Y Scale.Range:Minimum"), "YScale.Maximum"=100.0 ("Y Scale.Range:Maximum")) -> ()  [unwired: 2 in, 2 out]
              }
            }
          }
        }
        n2325 = disable-structure shown="Disabled" {
          frame Disabled {
            n2326 = case shown="True" {
              selector: _ -> [_ _]
              frame False {
              }
              frame True {
                n2327 = local read "zflag 2"() -> (w3138:dbl)
                n2328 = local read "yflag"() -> (w3140:dbl)
                n2329 = Equal?(x=w3140, y=2.0 ("tflag")) -> (x = y?=w3142:bool)
                n2330 = Equal?(x=w3138, y=3.0 ("tflag")) -> (x = y?=w3141:bool)
                n2331 = And(x=w3142, y=w3141) -> (x .and. y?=w3136:bool)
                n2332 = case shown="True" w3136 {
                  frame False {
                  }
                  frame True {
                    w3167 = 0.0 ("zflag")
                    n2333 = local write "zflag"(w3167) -> ()
                    n2334 = local write "zflag 2"(w3167) -> ()
                    n2335 = Delete(path (use dialog)=path "C:/LAB-IQ-NXT/WO 2449 TT.sig" ("file path (dialog if empty)")) -> (deleted path=w3166:path)  [unwired: 4 in, 2 out]
                    n2336 = Delete(path (use dialog)=path "C:/LAB-IQ-NXT/WO 2449 TRH.sig" ("file path (dialog if empty)")) -> (deleted path=w3161:path)  [unwired: 4 in, 2 out]
                    n2337 = local read "SEN.RUN HRS"() -> (w3153:dbl)
                    n2338 = local read "SENSOR TIME"() -> (w3151:dbl)
                    n2339 = call <vilib>:"compatOverwrite.vi"("overwrite (F)"=TRUE) -> ("overwrite?"=w3143:T30)
                    n2340 = call <vilib>:"compatOverwrite.vi"("overwrite (F)"=TRUE) -> ("overwrite?"=w3147:T30)
                    n2341 = local read "Total No. of Tests"() -> (w3154:dbl)
                    n2342 = Add(x=w3151, y=w3153) -> (x+y=w3152:dbl)
                    "SEN.RUN HRS" <- w3152
                    n2343 = Open/Create/Replace File(file path (use dialog)=w3166, operation (0:open)=w3143) -> (refnum out=w3144:refnum<file>, error out=w3145:errorcluster)  [unwired: 4 in, 1 out]
                    n2344 = Open/Create/Replace File(file path (use dialog)=w3161, operation (0:open)=w3147) -> (refnum out=w3148:refnum<file>, error out=w3149:errorcluster)  [unwired: 4 in, 1 out]
                    n2345 = Deny Access(4:w3145, 6:T28."deny none" ("deny mode (2)"), 7:w3144) -> (3:w3165:refnum<file>)  [unwired: 1 out]
                    n2346 = Deny Access(4:w3149, 6:T28."deny none" ("deny mode (2)"), 7:w3148) -> (3:w3157:refnum<file>)  [unwired: 1 out]
                    n2347 = Number To Decimal String(number=w3154) -> (decimal integer string=w3162:string)  [unwired: 1 in]
                    n2348 = Number To Decimal String(number=w3152) -> (decimal integer string=w3158:string)  [unwired: 1 in]
                    n2349 = Write to Binary File(file (use dialog)=w3165, data=w3162, 5:FALSE ("prepend array or string size? (T)")) -> ()  [unwired: 3 in, 3 out]
                    n2350 = Write to Binary File(file (use dialog)=w3157, data=w3158, 5:FALSE ("prepend array or string size? (T)")) -> ()  [unwired: 3 in, 3 out]
                  }
                }
              }
            }
          }
          frame Enabled {
          }
        }
        n2351 = local read "RUN"() -> (w3065:bool)
        n2352 = local read "run replace"() -> (w3069:bool)
        n2353 = local read "run replace"() -> (w3068:bool)
        n2354 = case shown="True" w3065 {
          frame False {
            n2355 = local write "run replace"(FALSE ("run replace")) -> ()
          }
          frame True {
            "run replace" <- TRUE ("run replace")
          }
        }
        n2356 = local read "RUN"() -> (w3073:bool)
        n2357 = local read "Set Temp"() -> (w3035:dbl)
        n2358 = local read "SetTemp"() -> (w3037:dbl)
        n2359 = case shown="False" w3073 {
          tunnel: [FALSE ("TEST RUNNING") TRUE ("TEST RUNNING")] -> w3072
          frame False {
            w3256 = 0.0 ("Flag")
            n2360 = local write "Elapsed time"(0.0 ("elapsedtime")) -> ()
            n2361 = local write "Time Remaining"(w3256) -> ()
            n2362 = local write "Flag"(w3256) -> ()
            n2363 = local write "Remaining Time"(w3256) -> ()
          }
          frame True {
            n2364 = local write "Flag"(10.0 ("Flag")) -> ()
          }
        }
        n2365 = case shown="False" w3069 {
          frame False {
            n2366 = local read "zflag"() -> (→"zflag 2":dbl)
            n2367 = local write "yflag"(2.0 ("tflag")) -> ()
            n2368 = local write "FLAG 4"(0.0 ("FLAG")) -> ()
          }
          frame True {
            n2369 = local write "yflag"(1.0 ("tflag")) -> ()
            n2370 = local write "zflag"(3.0 ("zflag")) -> ()
          }
        }
        n2371 = local read "acq 2"() -> (w3067:bool)
        n2372 = local read "AIR TEMP"() -> (w3030:dbl)
        n2373 = local read "Amb temp"() -> (w3034:dbl)
        n2374 = case shown="True" "Save & Continue" {
          frame False {
          }
          frame True {
            "acq 2" <- TRUE ("acq 2")
          }
        }
        n2375 = local read "Set Rh"() -> (w3036:dbl)
        n2376 = Add(x=w3037, y=w3062) -> (x+y=w3063:dbl)
        n2377 = Subtract(x=w3037, y=w3062) -> (x-y=w3064:dbl)
        n2378 = Add(x=w3035, y=w3056) -> (x+y=w3057:dbl)
        n2379 = Subtract(x=w3035, y=w3056) -> (x-y=w3058:dbl)
        n2380 = And(x=w3067, y=w3068) -> (x .and. y?=w3066:bool)
        n2381 = Greater Or Equal?(x=w3030, y=15.0) -> (x >= y?=w3031:bool)
        "powstat" <- w3031
        n2382 = local read "Humidity ( %RH )"() -> (w3033:dbl)
        n2383 = case shown="True" "Save & Continue" {
          frame False {
          }
          frame True {
            n2384 = while {
              tunnel: "0123456789abcdefghijklmnopqrstuvwxyzABCDEFGHIJKLMNOPQRSTUVWXYZ" ("string 2") -> [w3227]
              shift-right: [w3225] -> w3220
              shift-left: "" -> [w3224]
              i -> [w3234]
              stop <- w3233 stop-if-true
              n2385 = Random Number (0-1)() -> (number: 0 to 1=w3228:dbl)
              n2386 = Multiply(x=w3228, y=62.0) -> (x*y=w3230:dbl)
              n2387 = Decrement(x="Length") -> (x-1=w3223:i16)
              n2388 = To Word Integer(number=w3230) -> (16bit integer=w3231:i16)
              n2389 = String Subset(string=w3227, offset (0)=w3231, length (rest)=1 ("length (rest)")) -> (substring=w3226:string)
              n2390 = Greater Or Equal?(x=w3234, y=w3223) -> (x >= y?=w3233:bool)
              n2391 = Concatenate Strings(w3226, w3224) -> (w3225:string)
            }
            n2392 = local write "UUID"(w3220) -> ()
          }
        }
        n2393 = In Range and Coerce(upper limit=w3063, x=w3034, lower limit=w3064) -> (In Range?=w3053:bool)  [unwired: 1 out]
        n2394 = Add(x=w3036, y=w3061) -> (x+y=w3060:dbl)
        n2395 = Subtract(x=w3036, y=w3061) -> (x-y=w3059:dbl)
        n2396 = local read "TEMP"() -> (w3032:dbl)
        n2397 = case shown="True" "Save & Continue" {
          frame False {
          }
          frame True {
            n2398 = local read "Operator ID"() -> (w3551:string)
            n2399 = local read "FILE"() -> (w3557:string)
            n2400 = String Length(string=w3557) -> (length=w3555:i32)
            n2401 = String Length(string=w3551) -> (length=w3552:i32)
            n2402 = Greater?(x=w3555, y=0) -> (0:w3554:bool)
            n2403 = Greater?(x=w3552, y=0) -> (0:w3550:bool)
            n2404 = And(x=w3554, y=w3550) -> (x .and. y?=w3549:bool)
            n2405 = case shown="True" w3549 {
              frame False {
                n2406 = stacked-sequence {
                  frame #0 {
                    n2407 = One Button Dialog(message="Please Enter a File Name and Operator ID to save data !", button name ("OK")="Ok") -> ()  [unwired: 1 out]
                  }
                  frame #1 {
                    n2408 = local write "Save & Continue"(FALSE ("OK Button")) -> ()
                  }
                }
                n2409 = local write "Save & Continue"(FALSE ("OK Button")) -> ()
              }
              frame True {
                n2410 = stacked-sequence {
                  frame #0 {
                    n2411 = local read "FILE"() -> (w3563:string)
                    n2412 = call "file check.vi"("file name in"=w3563) -> ("file name out"=w3562:string)  [unwired: 9 in, 1 out]
                    n2413 = call <vilib>:"Application Directory.vi"() -> ("Application Directory"=w3573:path)
                    n2414 = Build Path(base path=w3573, name or relative path="data") -> (appended path=w3572:path)
                    n2415 = call <vilib>:"Trim Whitespace.vi"("string"=w3562) -> ("trimmed string"=w3570:string)  [unwired: 1 in]
                    n2416 = call <vilib>:"Trim Whitespace.vi"("string"=w3562) -> ("trimmed string"=w3571:string)  [unwired: 1 in]
                    n2417 = List Folder(path=w3572) -> (folder names=w3568:string[])  [unwired: 3 in, 3 out]
                    n2418 = Match Pattern(string=w3570, regular expression="_(") -> (before substring=w3567:string)  [unwired: 1 in, 3 out]
                    n2419 = for {
                      tunnel: w3568 -> [w3582] mode=indexing
                      tunnel: w3567 -> [w3580]
                      shift-right: [w3578] -> w3565
                      shift-left: bool[] [] -> [w3579]
                      n2420 = Match Pattern(string=w3582, regular expression="_(") -> (before substring=w3581:string)  [unwired: 1 in, 3 out]
                      n2421 = Equal?(x=w3581, y=w3580) -> (x = y?=w3577:bool)
                      n2422 = case shown="True" w3577 {
                        tunnel: w3577 -> [_ w3585]
                        tunnel: w3579 -> [w3584 w3587]
                        tunnel: [w3584 w3586] -> w3578
                        frame False {
                        }
                        frame True {
                          n2423 = Insert Into Array(array=w3587, new element=w3585) -> (w3586:bool[])  [unwired: 1 in]
                        }
                      }
                    }
                    n2424 = Equal?(x=w3568, y=w3567) -> (x = y?=w3576:bool[])
                    n2425 = Or Array Elements(Boolean array=w3576) -> (logical OR=w3575:bool)
                    n2426 = Array Size(array=w3565) -> (size(s)=w3564:i32)
                    n2427 = case shown="True" w3575 {
                      tunnel: w3571 -> [_ w3595]
                      tunnel: w3564 -> [_ w3588]
                      frame False {
                      }
                      frame True {
                        n2428 = Number To Decimal String(number=w3588) -> (decimal integer string=w3591:string)  [unwired: 1 in]
                        n2429 = Search/Split String(string=w3595, search string/char (-)="_(" ("regular expression")) -> (substring before match=w3593:string)  [unwired: 1 in, 2 out]
                        n2430 = Concatenate Strings(w3593, "_(" ("regular expression"), w3591, ")" ("regular expression")) -> (w3589:string)
                        n2431 = local write "FILE"(w3589) -> ()
                      }
                    }
                  }
                  frame #1 {
                    w3597 = 0.0
                    w3610 = cluster{"y":dbl, dbl, "y":dbl}[] [] ("History Data")
                    w3611 = FALSE ("Heater Button")
                    (unwired) ")!" ("string")
                    (unwired) ")" ("string")
                    w3609 = dbl[] [] ("History Data")
                    w3615 = "\r"
                    # "C:\\WinDucom\\Data\\"
                    # "C:\\LAB-IQ-NXT\\data"
                    n2432 = local write "Humidity ( %RH )"(w3597) -> ()
                    n2433 = local write "Frequency ( Hz )"(w3597) -> ()
                    n2434 = local write "Stroke 3"(w3597) -> ()
                    n2435 = local write "speedop"(0.0 ("PIDclk 2")) -> ()
                    n2436 = local write "Set Temp 2"(65.0 ("Set Temp 2")) -> ()
                    n2437 = local write "AIR TEMP"(w3597) -> ()
                    n2438 = local write "clk"(0.0 ("clk")) -> ()
                    n2439 = local write "Stroke 4"(w3597) -> ()
                    n2440 = local write "COF 2"(w3597) -> ()
                    n2441 = local write "TEMP"(w3597) -> ()
                    n2442 = local write "ecr 3"(w3597) -> ()
                    n2443 = local write "FF 3"(w3597) -> ()
                    n2444 = local write "FF 2"(w3597) -> ()
                    n2445 = property on="Humidity ( %RH )" class="WFChart (strict)"("History Data"=w3609) -> ()  [unwired: 2 in, 2 out]
                    n2446 = property on="Coefficient of Friction" class="WFChart (strict)"("History Data"=w3609) -> ()  [unwired: 2 in, 2 out]
                    n2447 = property on="Coefficient of Friction" class="WFChart (strict)"("History Data"=w3609) -> ()  [unwired: 2 in, 2 out]
                    n2448 = property on="Frictional Force ( N )" class="WFChart (strict)"("History Data"=w3609) -> ()  [unwired: 2 in, 2 out]
                    n2449 = property on="Electrical Contact Resistance ( % )" class="WFChart (strict)"("History Data"=w3609) -> ()  [unwired: 2 in, 2 out]
                    n2450 = property on="Electrical Contact Resistance ( % )" class="WFChart (strict)"("History Data"=w3609) -> ()  [unwired: 2 in, 2 out]
                    n2451 = property on="Temperature ( Deg C )" class="WFChart (strict)"("History Data"=w3609) -> ()  [unwired: 2 in, 2 out]
                    n2452 = property on="Frictional Force ( N )" class="WFChart (strict)"("History Data"=w3609) -> ()  [unwired: 2 in, 2 out]
                    n2453 = property on="Coefficient of Friction" class="WFChart (strict)"("History Data"=w3609) -> ()  [unwired: 2 in, 2 out]
                    n2454 = property on="Frictional Force ( N )" class="WFChart (strict)"("History Data"=w3609) -> ()  [unwired: 2 in, 2 out]
                    n2455 = property on="Electrical Contact Resistance ( % )" class="WFChart (strict)"("History Data"=w3609) -> ()  [unwired: 2 in, 2 out]
                    n2456 = property on="Temperature ( Deg C )" class="WFChart (strict)"("History Data"=w3609) -> ()  [unwired: 2 in, 2 out]
                    n2457 = property on="Humidity ( %RH )" class="WFChart (strict)"("History Data"=w3609) -> ()  [unwired: 2 in, 2 out]
                    n2458 = property on="Stroke ( mm )" class="WFChart (strict)"("History Data"=w3610) -> ()  [unwired: 2 in, 2 out]
                    n2459 = property on="Stroke ( mm )" class="WFChart (strict)"("History Data"=w3610) -> ()  [unwired: 2 in, 2 out]
                    n2460 = local write "Humidity"(w3611) -> ()
                    n2461 = local write "Heater Button"(w3611) -> ()
                    n2462 = local read "FILE"() -> (w3605:string)
                    n2463 = disable-structure shown="Enabled" {
                      disable-tunnel: [w3650 _] -> w3596
                      frame Enabled {
                        n2464 = local read "NORMAL LOAD"() -> (w3650:dbl)
                      }
                      frame Disabled {
                      }
                    }
                    n2465 = call "file check.vi"("file name in"=w3605) -> ("error out"=w3608:errorcluster, "file name out"=w3602:string)  [unwired: 9 in]
                    n2466 = call "FILE PATH CREATION.vi"("error in"=w3608, "FILE NAME :"=w3602) -> ("FILE OUT"=w3601:path)  [unwired: 8 in, 1 out]
                    n2467 = Concatenate Strings(w3602, ".dgf" ("Substring")) -> (w3607:string)
                    n2468 = Concatenate Strings(w3602, ".duf" ("Substring")) -> (w3603:string)
                    n2469 = Multiply(x=w3596, y=1.0) -> (x*y=w3629:dbl)
                    n2470 = Build Path(base path=w3601, name or relative path=w3607) -> (appended path=w3600:path)
                    n2471 = Build Path(base path=w3601, name or relative path=w3603) -> (appended path=w3599:path)
                    n2472 = Number To Fractional String(number=w3629, width (-)=i16 5, precision (6)=i16 2) -> (F-format string=w3637:string)  [unwired: 1 in]
                    n2473 = local read "Fuel Discription :"() -> (w3625:string)
                    n2474 = local read "Batch Ref Num :"() -> (w3613:string)
                    n2475 = Get Date/Time String(date format (0)=enum16{"short", "long", "abbreviated"}."short") -> (date string=w3648:string, time string=w3645:string)  [unwired: 2 in]
                    n2476 = local read "Remarks :"() -> (w3624:string)
                    n2477 = Concatenate Strings("Load :- " ("Substring"), w3637, " grams ," ("Substring")) -> (w3636:string)
                    n2478 = local read "String 41"() -> (w3616:string)
                    n2479 = Concatenate Strings(w3625) -> (w3626:string)
                    n2480 = Concatenate Strings(w3613) -> (w3612:string)
                    n2481 = Concatenate Strings("tested by") -> (w3620:string)
                    n2482 = Concatenate Strings("(" ("Substring"), w3648, ")" ("Substring"), w3645) -> (w3618:string)
                    "concatenated string" <- w3618
                    n2483 = Concatenate Strings(w3624, "," ("string")) -> (w3623:string)
                    n2484 = Concatenate Strings("  TIME;      COF;       STROKE;     AIR TEMP;  TEMP;  HUMIDITY;  ECR; PID-OUT; FREQUENCY" ("Substring"), "\r") -> (w3632:string)
